vi "LS330_MinMax.vi"(11 "Input Cluster":T2) -> (0 "Value Cluster":T1, 3 "output cluster":T2)   [LabVIEW 2021]
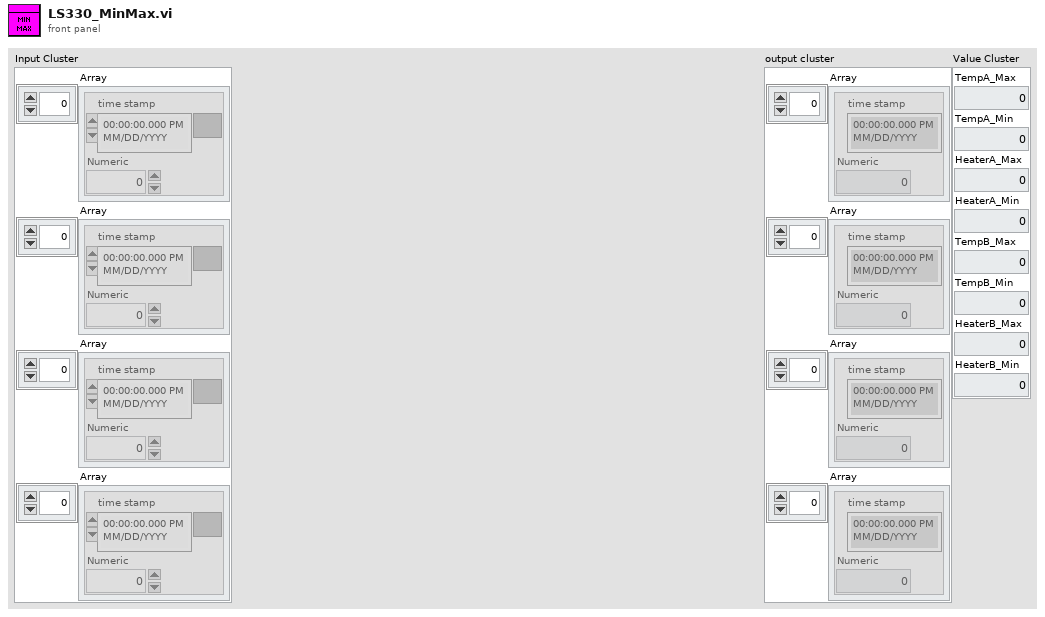
[diagram p1: front panel]
types:
  T1 = cluster{"TempA_Max":dbl, "TempA_Min":dbl, "HeaterA_Max":dbl, "HeaterA_Min":dbl, "TempB_Max":dbl, "TempB_Min":dbl, "HeaterB_Max":dbl, "HeaterB_Min":dbl}
  T2 = cluster{"Array":cluster{"time stamp":timestamp, "Numeric":dbl}[], "Array":cluster{"time stamp":timestamp, "Numeric":dbl}[], "Array":cluster{"time stamp":timestamp, "Numeric":dbl}[], "Array":cluster{"time stamp":timestamp, "Numeric":dbl}[]}
  T3 = cluster{cluster{"time stamp":timestamp, "Numeric":dbl}[], cluster{"time stamp":timestamp, "Numeric":dbl}[], cluster{"time stamp":timestamp, "Numeric":dbl}[], cluster{"time stamp":timestamp, "Numeric":dbl}[]}
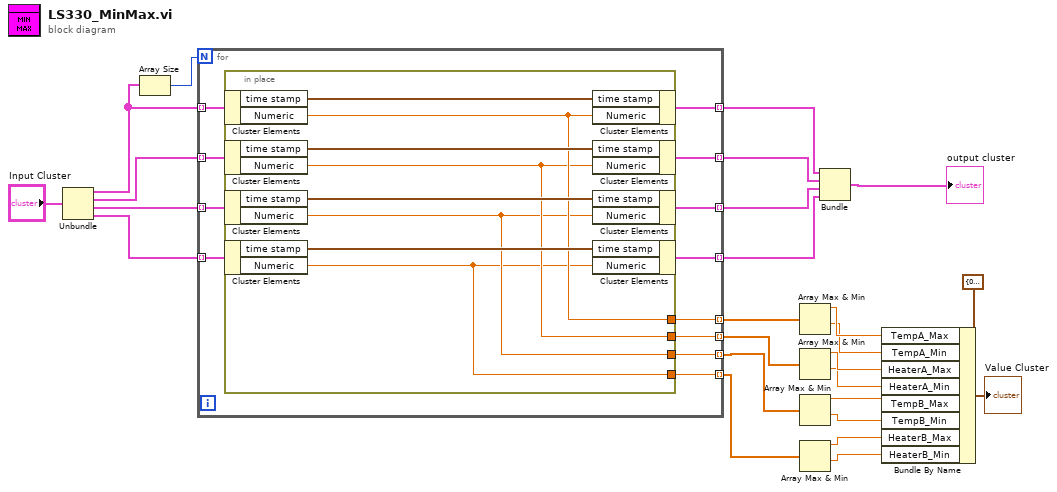
[diagram p0: block diagram]
diagram:
  n1 = Unbundle("Input Cluster") -> ("Array"=w21:cluster{"time stamp":timestamp, "Numeric":dbl}[], "Array"=w24:cluster{"time stamp":timestamp, "Numeric":dbl}[], "Array"=w23:cluster{"time stamp":timestamp, "Numeric":dbl}[], "Array"=w22:cluster{"time stamp":timestamp, "Numeric":dbl}[])
  n2 = Array Size(array=w21) -> (size(s)=w20:i32)
  n3 = for {
    N: w20 -> [_]
    tunnel: w21 -> [w37] mode=indexing
    tunnel: w24 -> [w36] mode=indexing
    tunnel: w23 -> [w35] mode=indexing
    tunnel: w22 -> [w34] mode=indexing
    tunnel: [w33] -> w15 mode=indexing
    tunnel: [w32] -> w14 mode=indexing
    tunnel: [w31] -> w13 mode=indexing
    tunnel: [w30] -> w12 mode=indexing
    tunnel: [w29] -> w19 mode=indexing
    tunnel: [w28] -> w18 mode=indexing
    tunnel: [w27] -> w17 mode=indexing
    tunnel: [w26] -> w16 mode=indexing
    n4 = in-place {
      in-place-border: [w41] -> w29
      in-place-border: [w40] -> w28
      in-place-border: [w39] -> w27
      in-place-border: [w38] -> w26
      n5 = in-place-cluster #1(w37) -> ("time stamp"=w45:timestamp, "Numeric"=w41:dbl)
      n6 = in-place-cluster #2(w36) -> ("time stamp"=w44:timestamp, "Numeric"=w40:dbl)
      n7 = in-place-cluster #3(w35) -> ("time stamp"=w42:timestamp, "Numeric"=w39:dbl)
      n8 = in-place-cluster #4(w34) -> ("time stamp"=w43:timestamp, "Numeric"=w38:dbl)
      n9 = in-place-cluster #1("time stamp"=w45, "Numeric"=w41) -> (w33:cluster{"time stamp":timestamp, "Numeric":dbl})
      n10 = in-place-cluster #2("time stamp"=w44, "Numeric"=w40) -> (w32:cluster{"time stamp":timestamp, "Numeric":dbl})
      n11 = in-place-cluster #3("time stamp"=w42, "Numeric"=w39) -> (w31:cluster{"time stamp":timestamp, "Numeric":dbl})
      n12 = in-place-cluster #4("time stamp"=w43, "Numeric"=w38) -> (w30:cluster{"time stamp":timestamp, "Numeric":dbl})
    }
  }
  n13 = Array Max & Min(array=w19) -> (max value=w9:dbl, min value=w8:dbl)  [unwired: 2 out]
  n14 = Array Max & Min(array=w18) -> (max value=w7:dbl, min value=w6:dbl)  [unwired: 2 out]
  n15 = Array Max & Min(array=w17) -> (max value=w5:dbl, min value=w4:dbl)  [unwired: 2 out]
  n16 = Array Max & Min(array=w16) -> (max value=w3:dbl, min value=w2:dbl)  [unwired: 2 out]
  n17 = Bundle(w15, w14, w13, w12) -> (→"output cluster":T3)  [unwired: 1 in]
  n18 = Bundle By Name(cluster=T1 {"TempA_Max"=0.0, "TempA_Min"=0.0, "HeaterA_Max"=0.0, "HeaterA_Min"=0.0, "TempB_Max"=0.0, "TempB_Min"=0.0, "HeaterB_Max"=0.0, "HeaterB_Min"=0.0} ("input cluster"), "TempA_Max"=w9, "TempA_Min"=w8, "HeaterA_Max"=w7, "HeaterA_Min"=w6, "TempB_Max"=w5, "TempB_Min"=w4, "HeaterB_Max"=w3, "HeaterB_Min"=w2) -> (→"Value Cluster":T1)
